vi "Create.vi"(8 "error in (no error)":errorcluster, 9 "Address [A2, A1, A0]":u8, 10 "I2C Bus":refnum<class "I2C Bus.lvclass">) -> (0 "error out":errorcluster, 3 "MCP23017":refnum<class "MCP23017.lvclass">)   [LabVIEW 2020, in "MCP23017.lvclass"]
uses:
  MCP23017.lvclass
  I2C Bus Interface/I2C Bus.lvclass
  MCP23017.lvclass/MCP23017.ctl
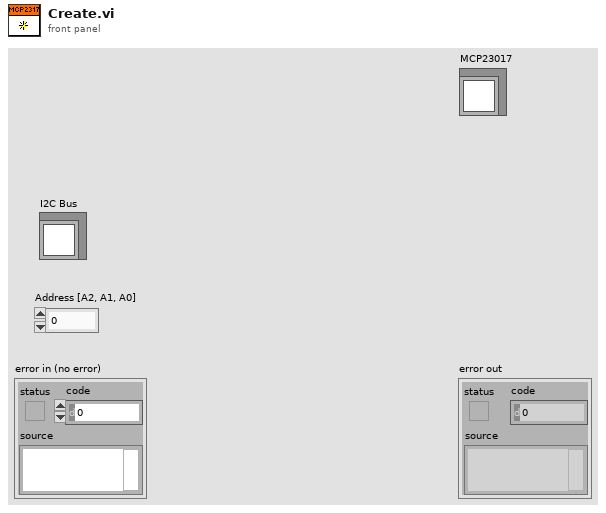
[diagram p1: front panel]
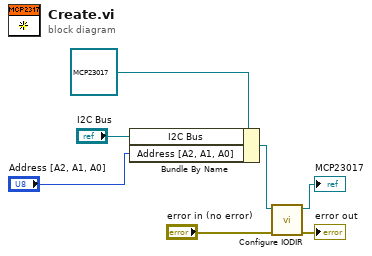
[diagram p0: block diagram]
diagram:
  n1 = Bundle By Name(cluster=refnum<class "MCP23017.lvclass"> refnum ("MCP23017"), "I2C Bus"="I2C Bus", "Address [A2, A1, A0]"="Address [A2, A1, A0]") -> (w5:refnum<class "MCP23017.lvclass">)
  n2 = call "Configure IODIR.vi"("error in (no error)"="error in (no error)", "MCP23017 In"=w5) -> ("error out"=→"error out":errorcluster, "MCP23017 Out"=→"MCP23017":refnum<class "MCP23017.lvclass">)  [unwired: 8 in]
